vi "SFID Get serial number.vi"(5 "COM port":refnum<visa-resource-name>) -> (0 "Error out":errorcluster, 1 "Serial number":u16, 2 "COM port out":refnum<visa-resource-name>)   [LabVIEW 2022 SP3]
uses:
  Ctls/SFID_Cmd.ctl
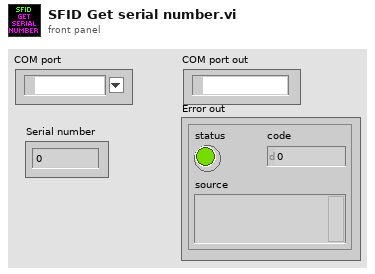
[diagram p1: front panel]
types:
  T1 = typedef "SFID_Cmd.ctl" = string
  T2 = enum16{"big-endian, network order", "native, host order", "little-endian"}
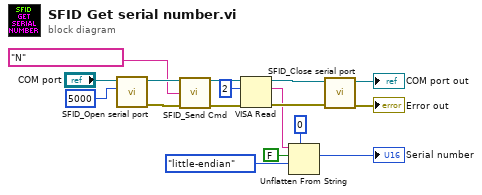
[diagram p0: block diagram]
diagram:
  n1 = call "SFID_Open serial port.vi"("timeout (ms)"=u32 5000, "VISA resource name"="COM port") -> ("Error out"=w12:errorcluster, "VISA resource name out"=w13:refnum<visa-resource-name>)  [unwired: 8 in]
  n2 = call "SFID_Send Cmd.vi"("Port"=w13, "Cmd"=T1 "N", "Error In"=w12) -> ("Port out"=w11:refnum<visa-resource-name>, "Error Out"=w10:errorcluster)  [unwired: 11 in]
  n3 = VISA Read(VISA resource name=w11, byte count=u32 2, error in (no error)=w10) -> (VISA resource name out=w6:refnum<visa-resource-name>, read buffer=w4:string, error out=w5:errorcluster)  [unwired: 1 out]
  "COM port out" <- w6
  n4 = Unflatten From String(type=u16 0 ("Serial number"), binary string=w4, data includes array or string size? (T)=FALSE, byte order (0:big-endian, network order)=T2."little-endian") -> (value=→"Serial number":u16)  [unwired: 1 in, 2 out]
  n5 = call "SFID_Close serial port.vi"("Error in"=w5, "VISA resource name"=w6) -> ("Error out"=→"Error out":errorcluster)  [unwired: 9 in]
